vi "Status Board.vi"() -> ()   [LabVIEW 2015]
panel:
  out "Status Board":string[][](table)
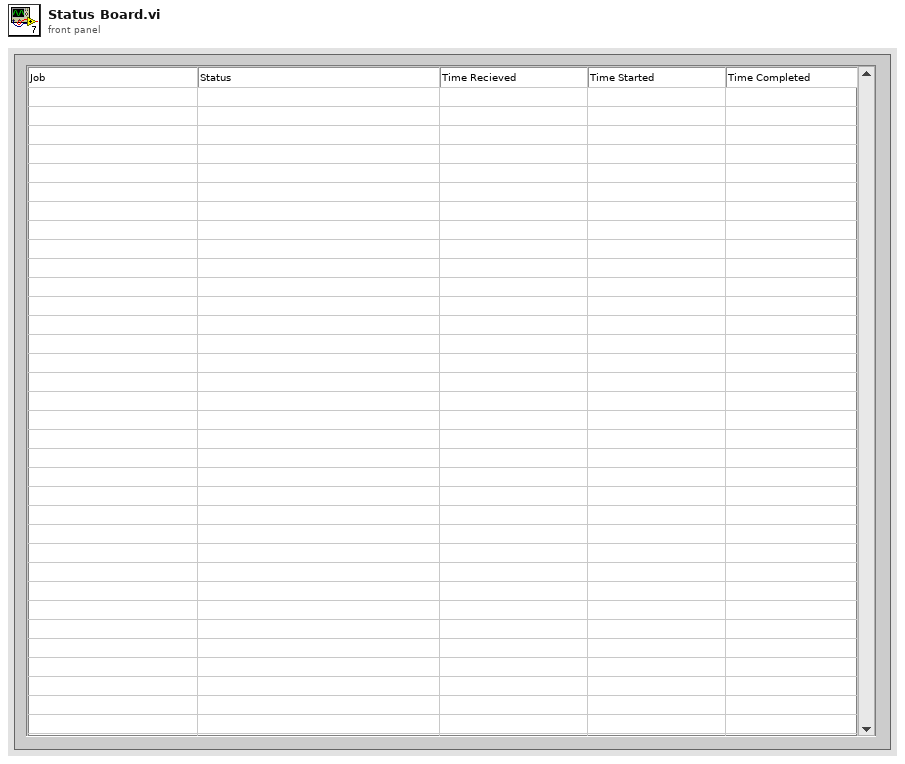
[diagram p1: front panel]
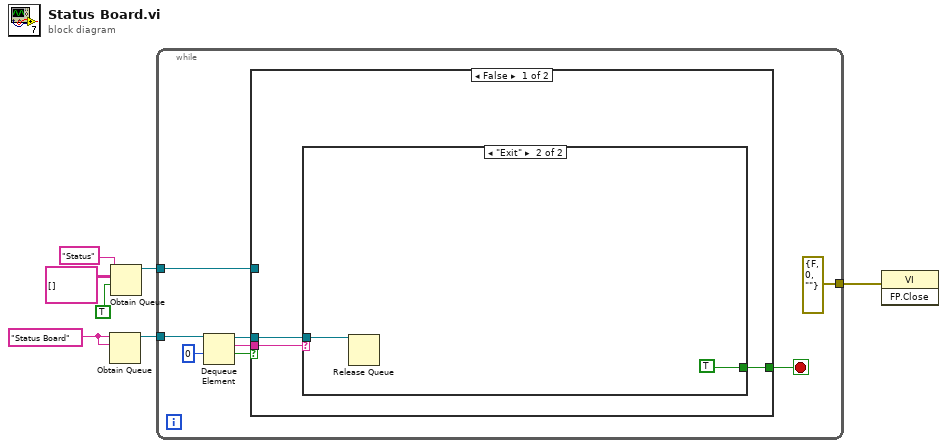
[diagram p0: block diagram]
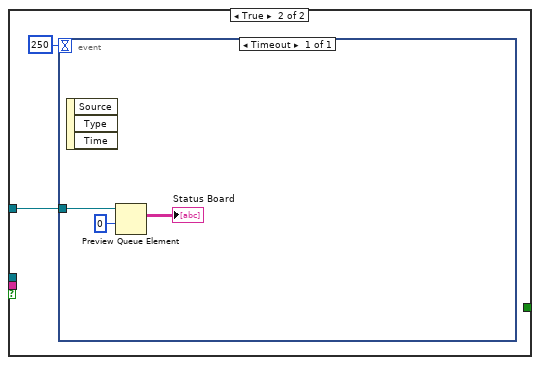
[diagram p3: hidden frame]
diagram:
  w3 = "Status Board" ("name (unnamed)")
  n1 = Obtain Queue(name (unnamed)=w3, element data type=w3) -> (queue out=w4:refnum<queue>)  [unwired: 3 in, 2 out]
  n2 = Obtain Queue(name (unnamed)="Status", element data type=string[][] [], create if not found? (T)=TRUE) -> (queue out=w5:refnum<queue>)  [unwired: 2 in, 2 out]
  n3 = while {
    tunnel: w5 -> [w15]
    tunnel: w4 -> [w14]
    tunnel: [errorcluster {"status"=FALSE, "code"=0, "source"=""} ("error in (no error)")] -> w1
    stop <- w9 stop-if-true
    n4 = Dequeue Element(queue=w14, timeout in ms (-1)=0) -> (queue out=w11:refnum<queue>, element=w10:string, timed out?=w12:bool)  [unwired: 1 in, 1 out]
    n5 = case shown="False" w12 {
      tunnel: w15 -> [_ w21]
      tunnel: w11 -> [w17 _]
      tunnel: w10 -> [w18 _]
      tunnel: [w16 _] -> w9
      frame False {
        n6 = case shown="\"Exit\"" w18 {
          tunnel: w17 -> [_ w20]
          tunnel: [_ TRUE] -> w16
          frame "", Default {
          }
          frame "Exit" {
            n7 = Release Queue(queue=w20) -> ()  [unwired: 2 in, 3 out]
          }
        }
      }
      frame True {
        n8 = event shown="[0] Timeout" {
          selector: _ -> [_]
          dyn-events: _ -> [_]
          timeout: 250 -> [_]
          tunnel: w21 -> [w24]
          event Timeout {
            n9 = event-data() -> ()  [unwired: 1 in, 3 out]
            n10 = Preview Queue Element(queue=w24, timeout in ms (-1)=0) -> (element=→"Status Board":string[][])  [unwired: 1 in, 3 out]
          }
        }
      }
    }
  }
  n11 = invoke class="VI" method="FP.Close"(error in=w1) -> ()  [unwired: 2 in, 3 out]
